vi "subDAQ_WaveformPorts.vi"(7 "DAQ ports":T1={"Lasers DO lines"=["Dev2/port0/line0", "Dev2/port0/line1", "Dev2/port0/line2", "Dev2/port0/line3", "Dev2/port0/line4", "Dev2/port0/line5"], "Lasers AO lines"=["Dev2/ao0", "Dev2/ao1", "Dev2/ao2", "Dev2/ao3", "Dev2/ao4", "Dev2/ao5"], "Patch AO line"="Dev1/ao1", "Patch AI lines 1"={"Patch scaled output"="Dev1/ai8", "Patch 10 V_m "="Dev1/ai0"}, "Camera timing DI"="Dev1/port0/line8", "Dev1 timing DO "="Dev1/port0/line9", "Dev1 trigger source"="/Dev1/PFI0", "Dev2 trigger source"="/Dev2/PFI0", "LED line"="Dev1/port0/line0", "Global Shutter line"="Dev2/port0/line6", "Patch AI lines 2"={"Cell capacitance"="Dev1/ai1", "Mode"="Dev1/ai2", "Frequency"="Dev1/ai3", "Gain"="Dev1/ai4"}}, 11 "Waveform channels":T2={"Lasers"=[FALSE, FALSE, FALSE, TRUE, FALSE, TRUE], "Patch"=TRUE, "Camera Output"=TRUE}) -> (3 "Waveform port selection":T3={"Lasers DO lines"=["Dev2/port0/line3", "Dev2/port0/line5"], "Lasers AO lines"=["Dev2/ao3", "Dev2/ao5"], "Patch AO line"="Dev1/ao0", "Patch AI lines"=["Dev1/ai0", "Dev1/ai8"], "Dev1 timing DO"="Dev1/port0/line1", "Camera timing DI"="Dev1/port0/line0", "Dev1 trigger source"="/Dev1/PFI0", "Dev2 trigger source"="/Dev2/PFI0"})   [LabVIEW 2015]
panel:
  # "637"
  # "561"
  # "532"
  # "488"
  # "405"
  # "Red"
  # "637"
  # "561"
  # "532"
  # "488"
  # "405"
  # "Red"
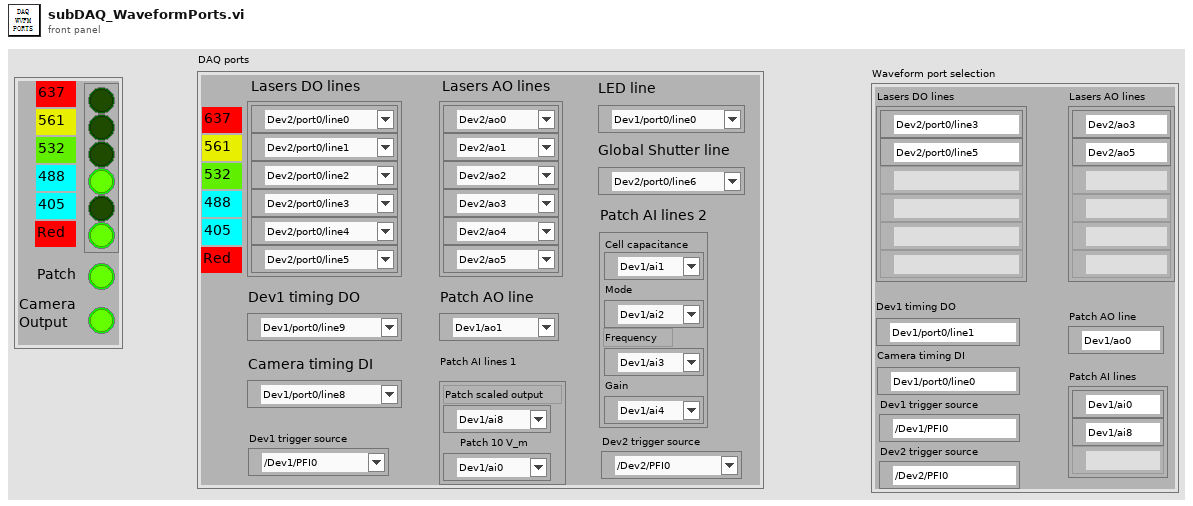
[diagram p1: front panel]
types:
  T1 = cluster{"Lasers DO lines":tag[], "Lasers AO lines":tag[], "Patch AO line":tag, "Patch AI lines 1":cluster{"Patch scaled output":tag, "Patch 10 V_m ":tag}, "Camera timing DI":tag, "Dev1 timing DO ":tag, "Dev1 trigger source":tag, "Dev2 trigger source":tag, "LED line":tag, "Global Shutter line":tag, "Patch AI lines 2":cluster{"Cell capacitance":tag, "Mode":tag, "Frequency":tag, "Gain":tag}}
  T2 = cluster{"Lasers":bool[], "Patch":bool, "Camera Output":bool}
  T3 = cluster{"Lasers DO lines":tag[], "Lasers AO lines":tag[], "Patch AO line":tag, "Patch AI lines":tag[], "Dev1 timing DO":tag, "Camera timing DI":tag, "Dev1 trigger source":tag, "Dev2 trigger source":tag}
  T4 = cluster{"Patch scaled output":tag, "Patch 10 V_m ":tag}
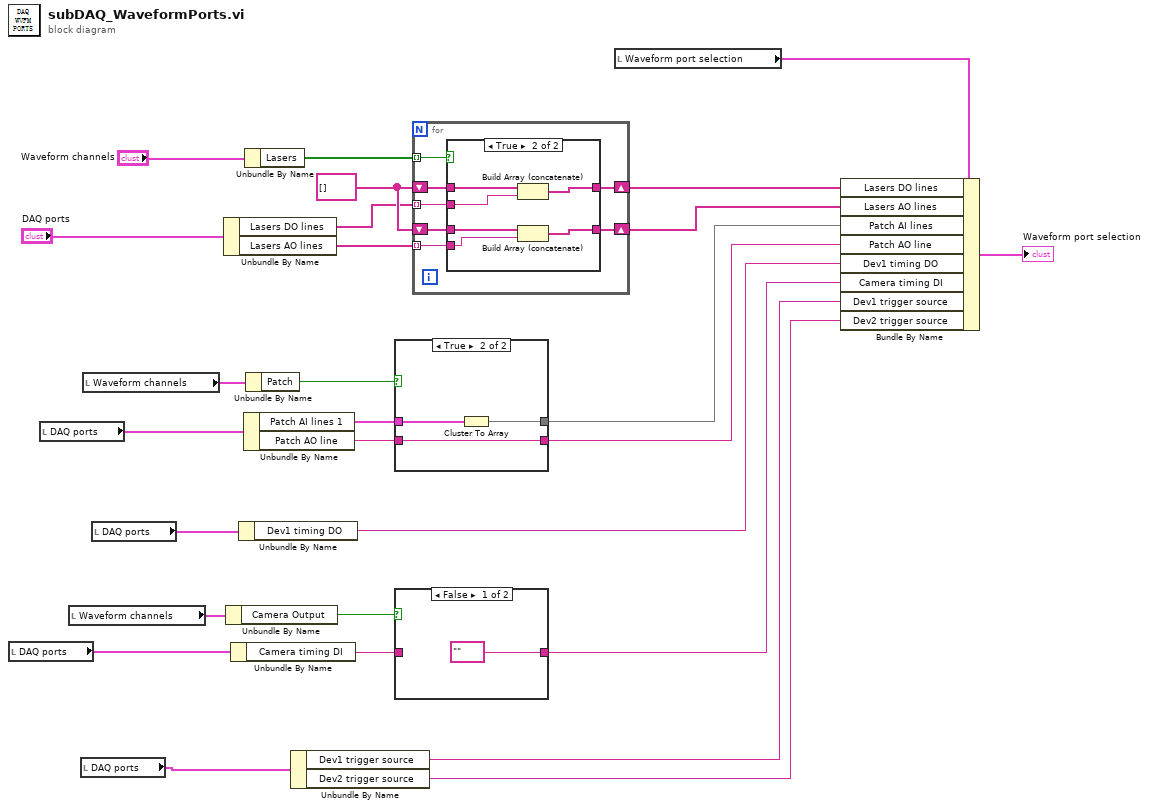
[diagram p0: block diagram]
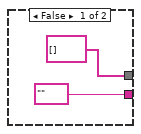
[diagram p3: hidden frame]
diagram:
  w26 = tag[] [] ("appended array")
  n1 = local read "DAQ ports"() -> (w2:T1)
  n2 = local read "DAQ ports"() -> (w4:T1)
  n3 = local read "Waveform channels"() -> (w10:T2)
  n4 = local read "DAQ ports"() -> (w1:T1)
  n5 = local read "Waveform channels"() -> (w11:T2)
  n6 = local read "DAQ ports"() -> (w3:T1)
  n7 = Unbundle By Name("DAQ ports") -> ("Lasers DO lines"=w16:tag[], "Lasers AO lines"=w15:tag[])
  n8 = Unbundle By Name(w10) -> ("Camera Output"=w17:bool)
  n9 = Unbundle By Name(w2) -> ("Camera timing DI"=w12:tag)
  n10 = Unbundle By Name(w3) -> ("Dev1 timing DO"=w8:tag)
  n11 = Unbundle By Name(w4) -> ("Patch AI lines 1"=w14:T4, "Patch AO line"=w13:tag)
  n12 = Unbundle By Name("Waveform channels") -> ("Lasers"=w27:bool[])
  n13 = Unbundle By Name(w11) -> ("Patch"=w21:bool)
  n14 = Unbundle By Name(w1) -> ("Dev1 trigger source"=w7:tag, "Dev2 trigger source"=w6:tag)
  n15 = case shown="True" w21 {
    tunnel: [tag[] [] ("AI lines") w32] -> w20
    tunnel: [tag "" ("Patch amplifier") w30] -> w19
    tunnel: w14 -> [_ w31]
    tunnel: w13 -> [_ w30]
    frame False {
    }
    frame True {
      n16 = Cluster To Array(cluster=w31) -> (array=w32:tag[])
    }
  }
  n17 = case shown="False" w17 {
    tunnel: [tag "" ("Patch amplifier") w34] -> w9
    tunnel: w12 -> [_ w34]
    frame False {
    }
    frame True {
    }
  }
  n18 = for {
    tunnel: w27 -> [w40] mode=indexing
    tunnel: w15 -> [w35] mode=indexing
    tunnel: w16 -> [w41] mode=indexing
    shift-right: [w39] -> w23
    shift-left: w26 -> [w38]
    shift-right: [w36] -> w22
    shift-left: w26 -> [w37]
    n19 = case shown="True" w40 {
      tunnel: w41 -> [_ w49]
      tunnel: [w43 w48] -> w39
      tunnel: w38 -> [w43 w47]
      tunnel: w37 -> [w42 w46]
      tunnel: [w42 w45] -> w36
      tunnel: w35 -> [_ w44]
      frame False {
      }
      frame True {
        n20 = Build Array (concatenate)(w47, w49) -> (w48:tag[])
        n21 = Build Array (concatenate)(w46, w44) -> (w45:tag[])
      }
    }
  }
  n22 = local read "Waveform port selection"() -> (w24:T3)
  n23 = Bundle By Name(cluster=w24, "Lasers DO lines"=w23, "Lasers AO lines"=w22, "Patch AI lines"=w20, "Patch AO line"=w19, "Dev1 timing DO"=w8, "Camera timing DI"=w9, "Dev1 trigger source"=w7, "Dev2 trigger source"=w6) -> (→"Waveform port selection":T3)
